vi "X Vision.vi"(2 "PID gain schedule for vision":T1(array[cluster])=[{"PID gains"={"proportional gain (Kc)"=0.005, "integral time (Ti, min)"=0.0, "derivative time (Td, min)"=0.003}, "max value"=5.0}, {"PID gains"={"proportional gain (Kc)"=0.0105, "integral time (Ti, min)"=0.0, "derivative time (Td, min)"=0.003}, "max value"=8.0}, {"PID gains"={"proportional gain (Kc)"=0.024, "integral time (Ti, min)"=0.0, "derivative time (Td, min)"=0.0}, "max value"=12.0}, {"PID gains"={"proportional gain (Kc)"=0.02, "integral time (Ti, min)"=0.0, "derivative time (Td, min)"=0.0}, "max value"=18.0}, {"PID gains"={"proportional gain (Kc)"=0.01, "integral time (Ti, min)"=0.0, "derivative time (Td, min)"=0.0}, "max value"=25.0}] {"max value" format="%.2f"; "PID gains"."derivative time (Td, min)" format="%.3f"; "PID gains"."integral time (Ti, min)" format="%.3f"; "PID gains"."proportional gain (Kc)" format="%.3f"}, 5 "Offset":dbl) -> (0 "X VISION":dbl=-0.020652084350585936)   [LabVIEW 2018]
uses:
  <vilib>/Rock Robotics/Network Tables/NT Read Number.vi
  <vilib>/addons/control/pid/pid.llb/PID Gain Schedule (DBL).vi
  <vilib>/addons/control/pid/pid.llb/PID (DBL).vi
  <vilib>/addons/control/pid/NI_PID_pid.lvlib
panel:
  out "tx":dbl=0.1304168701171875
  out "index out":i32
  in  "Reverse V":bool
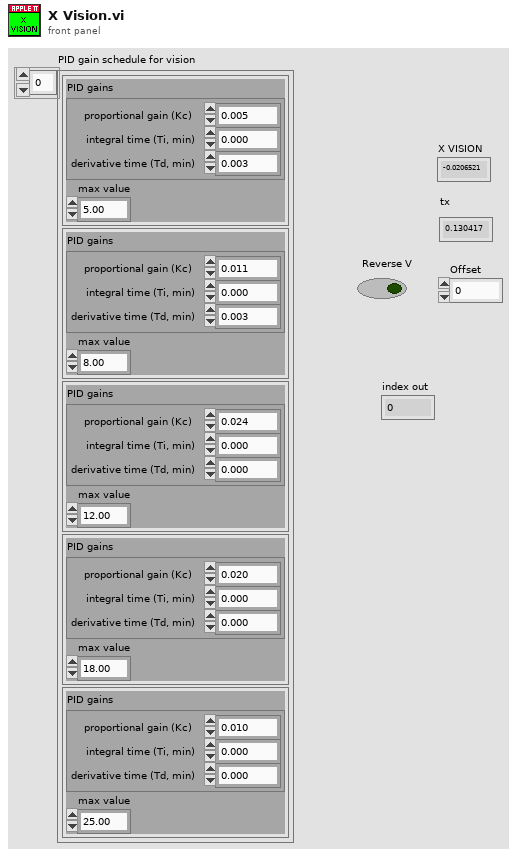
[diagram p1: front panel]
types:
  T1 = cluster{"PID gains":cluster{"proportional gain (Kc)":dbl, "integral time (Ti, min)":dbl, "derivative time (Td, min)":dbl}, "max value":dbl}[]
  T2 = cluster{"proportional gain (Kc)":dbl, "integral time (Ti, min)":dbl, "derivative time (Td, min)":dbl}
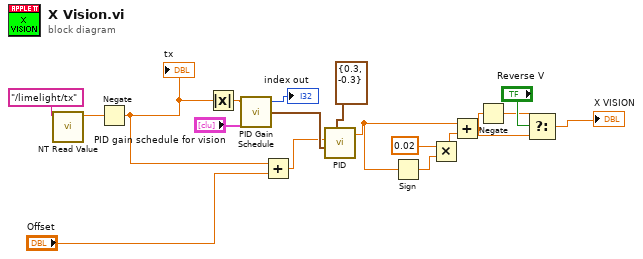
[diagram p0: block diagram]
diagram:
  n1 = call-poly <vilib>:"NT Read Value.vi"("Name"="/limelight/tx") -> ("Numeric"=w14:dbl)  [unwired: 9 in, 1 out]
  n2 = Negate(x=w14) -> (-x=w3:dbl)
  "tx" <- w3
  n3 = Absolute Value(x=w3) -> (abs(x)=w13:dbl)
  n4 = call-poly <vilib>:"PID Gain Schedule.vi"("PID gain schedule"="PID gain schedule for vision", "gain scheduling value"=w13) -> ("PID gains out"=w15:T2, "index out"=→"index out":i32)  [unwired: 2 in]
  n5 = Add(x=w3, y="Offset") -> (x+y=w4:dbl)
  n6 = call-poly <vilib>:"PID.vi"("output range"=cluster{"output high":dbl, "output low":dbl} {"output high"=0.3, "output low"=-0.3}, "PID gains"=w15, "process variable"=w4) -> ("output"=w9:dbl)  [unwired: 7 in, 1 out]
  n7 = Sign(1:w9) -> (0:w8:dbl)
  n8 = Multiply(x=0.02, y=w8) -> (x*y=w5:dbl)
  n9 = Add(x=w9, y=w5) -> (x+y=w6:dbl)
  n10 = Negate(x=w6) -> (-x=w16:dbl)
  n11 = Select(t=w16, s="Reverse V", f=w6) -> (s? t:f=→"X VISION":dbl)
